vi "Configure Filter.vi"(7 "Enable Sync Filter (F: Disable)":bool, 8 "error in (no error)":errorcluster, 9 "Low Pass Filter Slope (1: 12dB/oct)":u16(ring)=1 items=["6 dB/oct", "12 dB/oct", "18 db/oct", "24 dB/oct"], 10 "Time Constant (8: 100ms)":u16(ring)=8 items=["10 us", "30 us", "100 us", "300 us", "1 ms", "3 ms", "10 ms", "30 ms", "100 ms", "300 ms", "1 s", "3 s", "10 s", "30 s", "100 s", "300 s", "1 ks", "3 ks", "10 ks", "30 ks"], 11 "VISA resource name":refnum<visa-resource-name>) -> (0 "error out":errorcluster, 3 "VISA resource name out":refnum<visa-resource-name>)   [LabVIEW 2012, in "Stanford Research 830.lvlib"]
doc: "Configures the instrument's filter options.\n\n<B>Note:</B>\n\nThe Notch Filter is configured in <B>Configure Input Signal.vi</B>"
uses:
  <instrlib>/Stanford Research 830/Stanford Research 830.lvlib
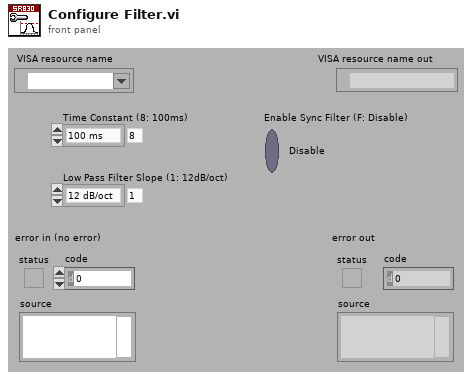
[diagram p1: front panel]
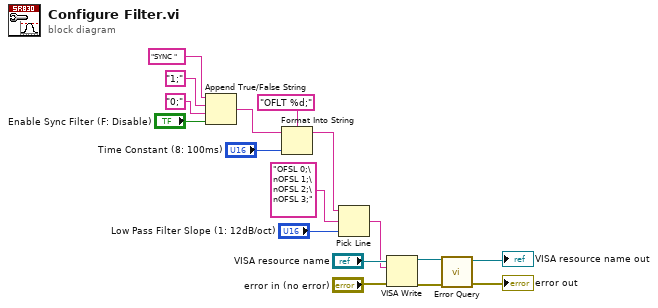
[diagram p0: block diagram]
diagram:
  n1 = Append True/False String(1:"Enable Sync Filter (F: Disable)", 2:"0;" ("false string"), 3:"1;" ("true string"), 4:"SYNC " ("string (\"\")")) -> (0:w9:string)
  n2 = Format Into String(format string="OFLT %d;", initial string=w9, "Time Constant (8: 100ms)") -> (resulting string=w7:string)  [unwired: 1 in, 1 out]
  n3 = Pick Line(string ("")=w7, multi-line string="OFSL 0;\nOFSL 1;\nOFSL 2;\nOFSL 3;", line index="Low Pass Filter Slope (1: 12dB/oct)") -> (output string=w5:string)
  n4 = VISA Write(VISA resource name="VISA resource name", write buffer=w5, error in (no error)="error in (no error)") -> (VISA resource name out=w4:refnum<visa-resource-name>, error out=w3:errorcluster)  [unwired: 1 out]
  n5 = call <instrlib>:"Error Query.vi"("error in (no error)"=w3, "VISA resource name"=w4) -> ("error out"=→"error out":errorcluster, "VISA resource name out"=→"VISA resource name out":refnum<visa-resource-name>)  [unwired: 7 in, 1 out]
